vi "MSI_Image_overlap.vi"() -> ()   [LabVIEW 2016]
uses:
  <vilib>/vision/NI_Vision_Development_Module.lvlib
panel:
  in  "Angle (degrees)":sgl format="%.2f"
  in  "Transparency":u8 max=80 step=1
  in  "stop":bool
  in  "Open":bool
  in  "Current rotation":sgl format="%.2f"
  out "Overlayed Image":T1(plugin-control)
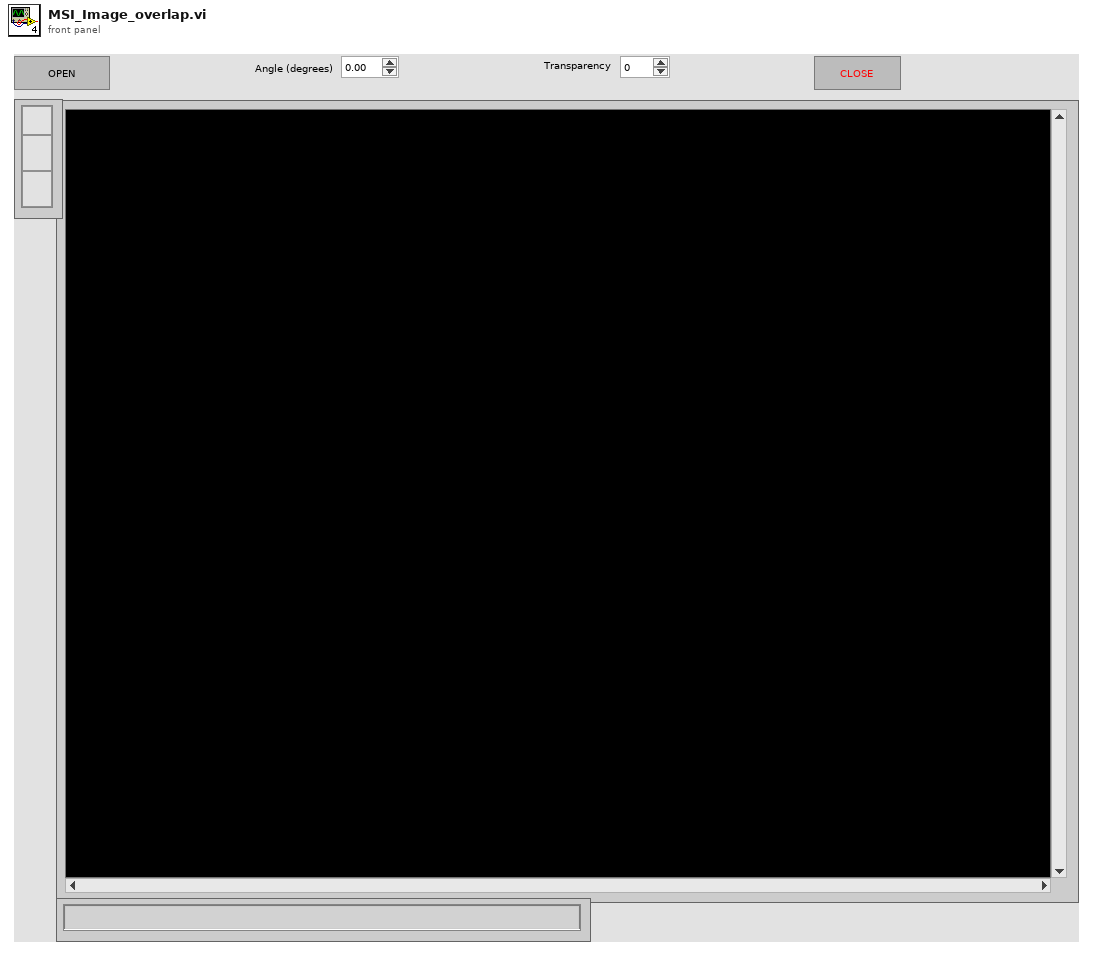
[diagram p1: front panel]
types:
  T1 = typedef "IMAQ Image.ctl" = refnum<image>
  T2 = cluster{"Blue or Luma":u8, "Green or Sat Plane":u8, "Red or Hue Plane":u8, "Alpha":u8}
  T3 = typedef "Image Type" = u32
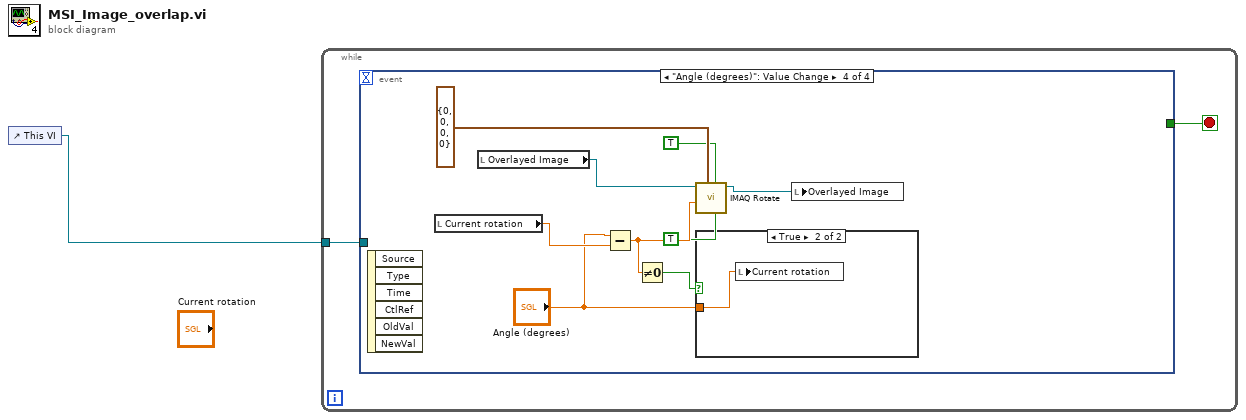
[diagram p0: block diagram]
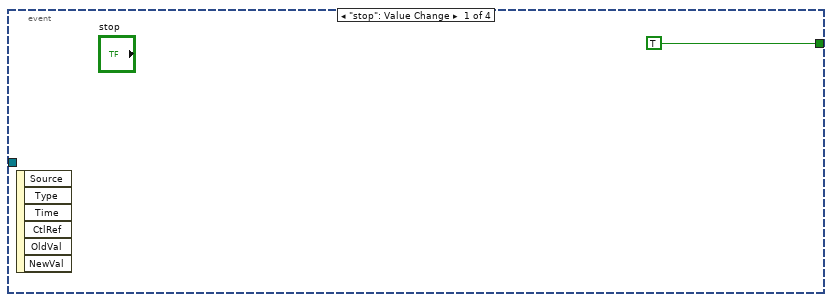
[diagram p2: hidden frame]
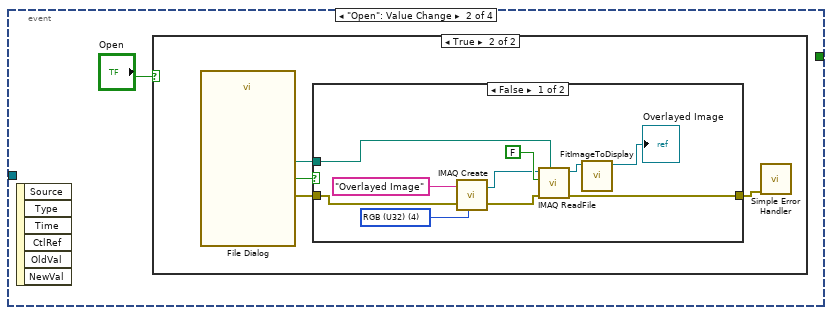
[diagram p3: hidden frame]
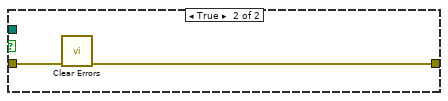
[diagram p5: hidden frame]
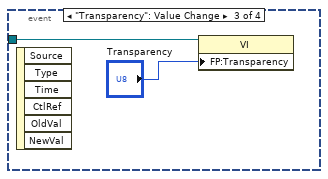
[diagram p6: hidden frame]
diagram:
  n1 = control-ref of="This VI"() -> (w1:refnum<vi>)
  n2 = while {
    tunnel: w1 -> [w2]
    stop <- w3 stop-if-true
    n3 = event shown="[3] \"Angle (degrees)\": Value Change" {
      selector: _ -> [_ _ _ _]
      dyn-events: _ -> [_ _ _ _]
      timeout: _ -> [_ _ _ _]
      tunnel: [TRUE ("stop") _ _ _] -> w3
      tunnel: w2 -> [_ _ w22 _]
      event "stop": Value Change {
        n4 = event-data() -> ()  [unwired: 1 in, 6 out]
      }
      event "Open": Value Change {
        n5 = event-data() -> ()  [unwired: 1 in, 6 out]
        n6 = case shown="True" "Open" {
          frame False {
          }
          frame True {
            n7 = call "File Dialog"() -> ("selected path"=w7:path, "cancelled"=w8:bool, "error out"=w9:errorcluster)  [unwired: 12 in, 1 out]
            n8 = case shown="False" w8 {
              tunnel: w7 -> [w19 _]
              tunnel: w9 -> [w10 w21]
              tunnel: [w16 w20] -> w6
              frame False {
                w15 = T3 4 items=["Grayscale (U8)", "Grayscale (I16)", "Grayscale (SGL)", "Complex (CSG)", "RGB (U32)", "HSL (U32)", "RGB (U64)", "Grayscale (U16)"] ("Image Type")
                n9 = call "IMAQ Create"("Image Name"="Overlayed Image", "Image Type"=w15, "error in (no error)"=w10) -> ("New Image"=w13:T1, "error out"=w11:errorcluster)  [unwired: 2 in]
                n10 = call "IMAQ ReadFile"("File Path"=w19, "error in (no error)"=w11, "Load Color Palette? (No)"=FALSE, "Image"=w13) -> ("error out"=w16:errorcluster, "Image Out"=w18:T1)  [unwired: 3 in, 3 out]
                n11 = call "FitImageToDisplay.vi"("Image"=w18) -> ("Image (dup)"=→"Overlayed Image":T1)  [unwired: 9 in]
              }
              frame True {
                n12 = call <vilib>:"Clear Errors.vi"("error in (no error)"=w21) -> ("error out"=w20:errorcluster)  [unwired: 5 in, 1 out]
              }
            }
            n13 = call <vilib>:"Simple Error Handler.vi"("error in (no error)"=w6) -> ()  [unwired: 4 in, 5 out]
          }
        }
      }
      event "Transparency": Value Change {
        n14 = event-data() -> ()  [unwired: 1 in, 6 out]
        n15 = property class="VI"(reference=w22, "FP:Transparency"="Transparency") -> ()  [unwired: 1 in, 2 out]
      }
      event "Angle (degrees)": Value Change {
        n16 = event-data() -> ()  [unwired: 1 in, 6 out]
        n17 = local read "Current rotation"() -> (w28:sgl)
        n18 = local read "Overlayed Image"() -> (w32:T1)
        n19 = Subtract(x="Angle (degrees)", y=w28) -> (x-y=w26:sgl)
        n20 = Not Equal To 0?(x=w26) -> (x != 0?=w25:bool)
        n21 = call "IMAQ Rotate"("Use Bilinear Interpolation"=TRUE, "Maintain Size"=TRUE, "Color Replace Value"=T2 {"Blue or Luma"=0, "Green or Sat Plane"=0, "Red or Hue Plane"=0, "Alpha"=0}, "Angle (degrees)"=w26, "Image Src"=w32) -> ("Image Dst Out"=w31:T1)  [unwired: 5 in, 1 out]
        n22 = case shown="True" w25 {
          tunnel: "Angle (degrees)" -> [_ w33]
          frame False {
          }
          frame True {
            n23 = local write "Current rotation"(w33) -> ()
          }
        }
        n24 = local write "Overlayed Image"(w31) -> ()
      }
    }
  }
